vi "Actor Core.vi"(8 "error in":errorcluster, 11 "State in":refnum<class "Drive Train.lvclass">) -> (0 "error out":errorcluster, 3 "Actor out":refnum<class "Actor.lvclass">)   [LabVIEW 2013, in "Virtual Systems.lvlib" / "Drive Train.lvlib" / "Drive Train.lvclass"]
doc: "(<B>Filename</B>: Actor Framework.lvlib:Actor.lvclass:Actor Core.vi)\n\nThis override invokes Entry.vi on the initial state, prior to calling the parent Actor Core. Adding this behavior to Actor Core (instead of an override of Pre Launch Init.vi) allows the initial state to launch a nested actor as part of its entry behavior.\n\nReceives messages to the actor, reacts to them, and initiates any error handling that may shut the actor down.\n\nDescendant classes may override this VI to append parallel tasks for the actor to complete while it handles messages. Overrides use the Call Parent Method node."
uses:
  Drive Train.lvclass
  <vilib>/ActorFramework/Actor/Actor.lvclass
  Robot/Logical Systems/Drive Train/Drive Train Class/Drive Train Status.ctl
  Robot/Logical Systems/Drive Train/Drive Train Class/Drive Train.lvclass
panel:
  in  "Drive Train Status":T1 {"Right Power Setpoint" min=-1.0 max=1.0 step=0.1 scale=-1.0..1.0; "Left Power Setpoint" min=-1.0 max=1.0 step=0.1 scale=-1.0..1.0; "Right Power" min=-1.0 max=1.0 step=0.1 scale=-1.0..1.0; "Left Power" min=-1.0 max=1.0 step=0.1 scale=-1.0..1.0}
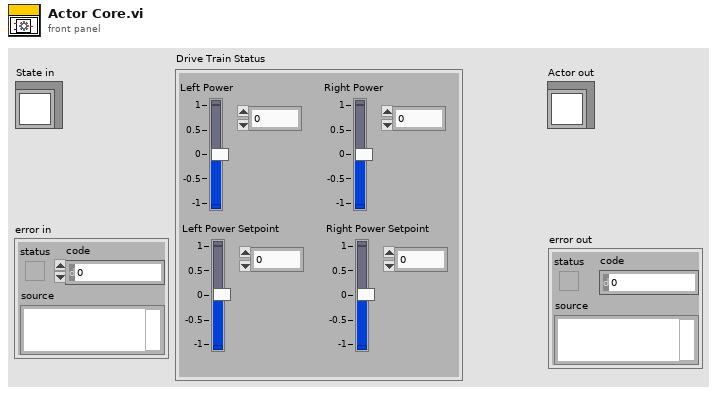
[diagram p1: front panel]
types:
  T1 = typedef "Logical Systems.lvlib/Drive Train.lvlib/Drive Train.lvclass/Drive Train Status.ctl" = cluster{"Left Power":dbl, "Right Power":dbl, "Left Power Setpoint":dbl, "Right Power Setpoint":dbl}
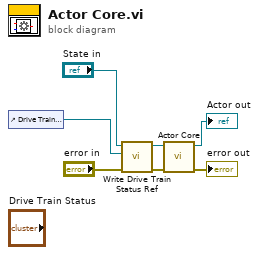
[diagram p0: block diagram]
diagram:
  n1 = control-ref of="Drive Train Status"() -> (w3:refnum<vi>)
  n2 = call-dynamic "Write Drive Train Status Ref.vi"("error in (no error)"="error in", "Drive Train Status Ref"=w3, "Drive Train in"="State in") -> ("error out"=w1:errorcluster, "Drive Train out"=w4:refnum<class "Drive Train.lvclass">)  [unwired: 7 in]
  n3 = call-parent "Actor Core.vi"("error in"=w1, "State in"=w4) -> ("error out"=→"error out":errorcluster, "Actor out"=→"Actor out":refnum<class "Actor.lvclass">)  [unwired: 8 in]
